vi "NaN Check.vi"(11 "Input":dbl[](array[numeric])) -> (3 "Output":dbl[](array[numeric]))   [LabVIEW 2017]
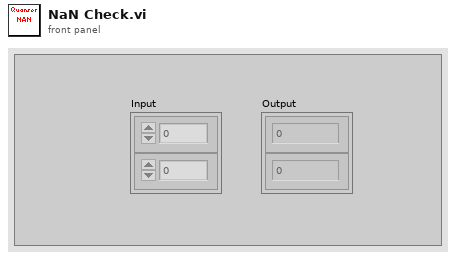
[diagram p1: front panel]
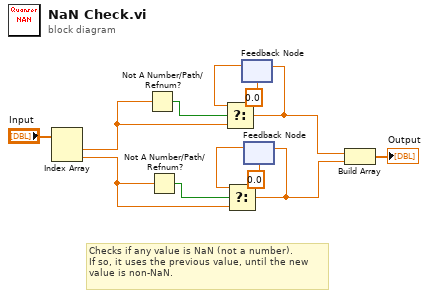
[diagram p0: block diagram]
diagram:
  # "Checks if any value is NaN (not a number).\nIf so, it uses the previous value, until the new \nvalue is non-NaN."
  n1 = Index Array(array="Input") -> (element #1=w3:dbl, element #2=w2:dbl)  [unwired: 2 in]
  n2 = Not A Number/Path/Refnum?(number/path/refnum=w3) -> (NaN/Path/Refnum?=w11:bool)
  n3 = Not A Number/Path/Refnum?(number/path/refnum=w2) -> (NaN/Path/Refnum?=w8:bool)
  n4 = feedback #1(0.0 ("Input")) -> (w12:dbl)
  n5 = Select(t=w12, s=w11, f=w3) -> (s? t:f=w6:dbl)
  n6 = feedback-in #1(w6) -> ()
  n7 = feedback #2(0.0 ("Input")) -> (w9:dbl)
  n8 = Select(t=w9, s=w8, f=w2) -> (s? t:f=w5:dbl)
  n9 = feedback-in #2(w5) -> ()
  n10 = Build Array(w6, w5) -> (→"Output":dbl[])
